vi "Create Chans.vi"(5 "New Section Name (none)":string, 6 "new section GUID (\"\":del prot)":string, 7 "Type":T3=enum."Output", 8 "error in (no error)":errorcluster, 10 "Channels":T2[](array[typedef]), 11 "Section Ptr":T1 format="%.0x") -> (0 "error out":errorcluster, 1 "new channel references":T1[](array[typedef]) format="%.0x", 2 "new section ref":T1=18446744073709551615 format="%.0x", 3 "Section Ptr dup":T1 format="%.0x")   [LabVIEW 2015, in "DCM System Explorer.lvlib"]
uses:
  DCM System Explorer.lvlib
  <vilib>/NI Veristand/Custom Device API/Custom Device Item Ref.ctl
  <vilib>/NI Veristand/Custom Device API/Custom Device Channel Type.ctl
  Shared/Types/Channel.ctl
  <vilib>/NI Veristand/Custom Device API/Custom Device Channel.ctl
  Shared/DCM Constants and GUIDs.vi
  <vilib>/NI VeriStand/Custom Device API/Custom Device API.lvlib
  DCM Shared.lvlib
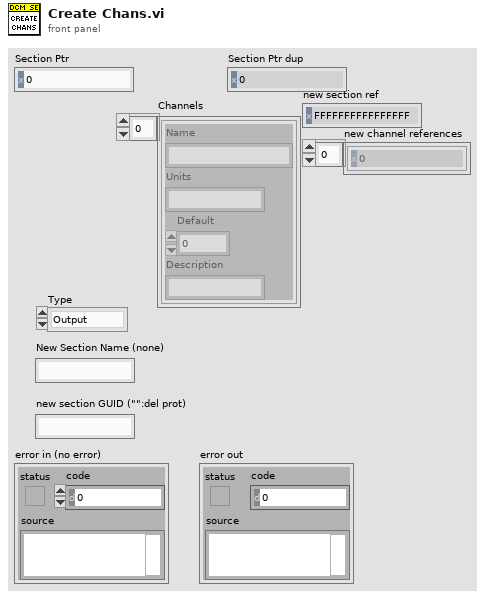
[diagram p1: front panel]
types:
  T1 = typedef "Custom Device API.lvlib/Custom Device Item Ref.ctl" = u64
  T2 = typedef "DCM Shared.lvlib/Channel.ctl" = cluster{"Name":string, "Units":string, "Default":dbl, "Description":string}
  T3 = typedef "Custom Device API.lvlib/Custom Device Channel Type.ctl" = enum16{"Input", "Output"}
  T4 = typedef "Custom Device API.lvlib/Custom Device Channel.ctl" = cluster{"Type":T3, "Units":string, "Default Value":dbl, "Faultable":bool, "Scalable":bool}
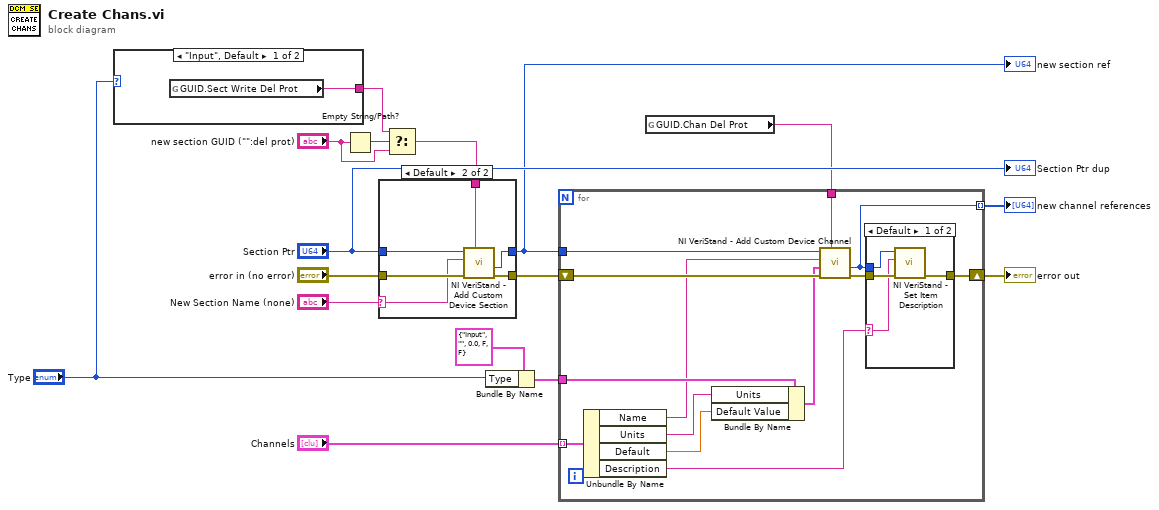
[diagram p0: block diagram]
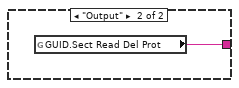
[diagram p2: hidden frame]
diagram:
  n1 = case shown="\"Input\", Default" "Type" {
    tunnel: [w17 w18] -> w1
    frame "Input", Default {
      n2 = global read "DCM Constants and GUIDs.vi" "GUID.Sect Write Del Prot"() -> (w17:string)
    }
    frame "Output" {
      n3 = global read "DCM Constants and GUIDs.vi" "GUID.Sect Read Del Prot"() -> (w18:string)
    }
  }
  n4 = Empty String/Path?(string/path="new section GUID (\"\":del prot)") -> (empty?=w7:bool)
  n5 = Select(t=w1, s=w7, f="new section GUID (\"\":del prot)") -> (s? t:f=w5:string)
  n6 = case shown="Default" "New Section Name (none)" {
    selector: "New Section Name (none)" -> [_ w22]
    tunnel: "error in (no error)" -> [w20 w26]
    tunnel: "Section Ptr" -> [w19 w25]
    tunnel: [w20 w24] -> w11
    tunnel: [w19 w23] -> w10
    tunnel: w5 -> [_ w21]
    frame "" {
    }
    frame Default {
      n7 = call <vilib>:"NI VeriStand - Add Custom Device Section.vi"("GUID (Default Section)"=w21, "error in (no error)"=w26, "Section Name"=w22, "Parent Ref in"=w25) -> ("error out"=w24:errorcluster, "Section Ptr"=w23:T1)  [unwired: 4 in, 2 out]
    }
  }
  "new section ref" <- w10
  n8 = Bundle By Name(cluster=T4 {"Type"=enum."Input", "Units"="", "Default Value"=0.0, "Faultable"=FALSE, "Scalable"=FALSE} ("Channel"), "Type"="Type") -> (w12:T4)
  n9 = global read "DCM Constants and GUIDs.vi" "GUID.Chan Del Prot"() -> (w3:string)
  n10 = for {
    tunnel: w10 -> [w38]
    shift-right: [w34] -> w15
    shift-left: w11 -> [w39]
    tunnel: w12 -> [w37]
    tunnel: w3 -> [w35]
    tunnel: "Channels" -> [w32] mode=indexing
    tunnel: [w27] -> w4 mode=indexing
    n11 = Unbundle By Name(w32) -> ("Name"=w31:string, "Units"=w30:string, "Default"=w29:dbl, "Description"=w28:string)
    n12 = Bundle By Name(cluster=w37, "Units"=w30, "Default Value"=w29) -> (w36:T4)
    n13 = call <vilib>:"NI VeriStand - Add Custom Device Channel.vi"("GUID (Default Channel)"=w35, "error in (no error)"=w39, "Channel"=w36, "Channel Name"=w31, "Parent Ref in"=w38) -> ("error out"=w33:errorcluster, "Channel Ref"=w27:T1)  [unwired: 3 in, 2 out]
    n14 = case shown="Default" w28 {
      selector: w28 -> [w40 _]
      tunnel: [w42 w44] -> w34
      tunnel: w33 -> [w43 w44]
      tunnel: w27 -> [w41 _]
      frame Default {
        n15 = call <vilib>:"NI VeriStand - Set Item Description.vi"("error in (no error)"=w43, "Description"=w40, "Item Ref in"=w41) -> ("error out"=w42:errorcluster)  [unwired: 6 in, 2 out]
      }
      frame "" {
      }
    }
  }
  "error out" <- w15
  "new channel references" <- w4
  "Section Ptr dup" <- "Section Ptr"
